vi "Is Transmit Ready.vi"(6 "Buffer size":i32=16384 format="0x%x (0d%d)", 8 "error in (no error)":errorcluster, 10 "Samples to transmit":i32=1024, 11 "Spectrum Recorder too in":refnum<class "Spectrum Recorder too.lvclass">) -> (0 "error out":errorcluster, 1 "Unused buffer":i32, 2 "Transmit Ready":bool, 3 "Spectrum Recorder too out":refnum<class "Spectrum Recorder too.lvclass">)   [LabVIEW 2016, in "Spectrum Recorder too.lvclass"]
uses:
  Spectrum Recorder too.lvclass
  Read RP transceiver.vi
  Write RP transceiver.vi
  NHMFL_Core/Libraries/Red Pitaya/RP Core/RP Transceiver/RP Transceiver.lvclass
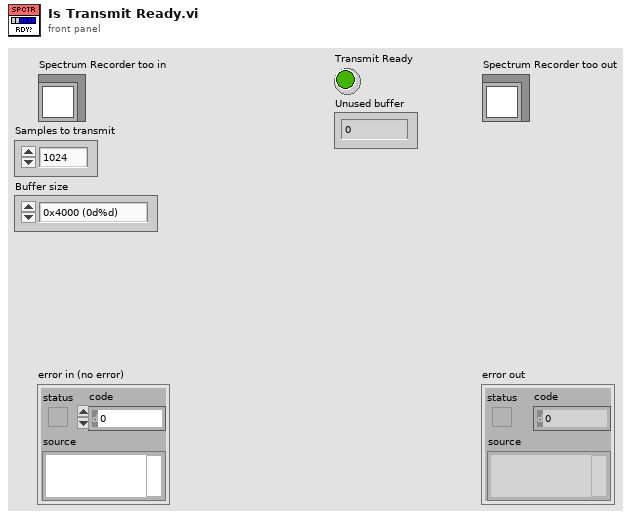
[diagram p1: front panel]
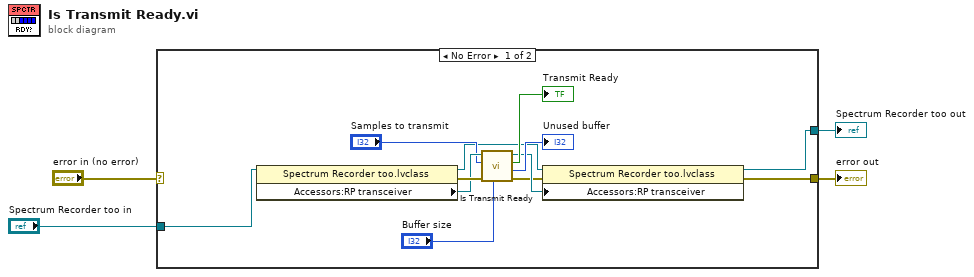
[diagram p0: block diagram]
diagram:
  n1 = case shown="No Error" "error in (no error)" {
    selector: "error in (no error)" -> [_ w18]
    tunnel: [w5 w18] -> w3
    tunnel: [w8 w17] -> w1
    tunnel: "Spectrum Recorder too in" -> [w15 w17]
    frame No Error {
      n2 = property class="Spectrum Recorder too.lvclass"(reference=w15) -> (reference out=w9:refnum<class "Spectrum Recorder too.lvclass">, error out=w16:errorcluster, "Accessors:RP transceiver"=w14:refnum<class "RP Transceiver.lvclass">)  [unwired: 1 in]
      n3 = call-dynamic "Is Transmit Ready.vi"("Buffer size"="Buffer size", "error in (no error)"=w16, "Samples to transmit"="Samples to transmit", "RP Instrument in"=w14) -> ("error out"=w6:errorcluster, "Unused buffer"=→"Unused buffer":i32, "Transmit Ready"=→"Transmit Ready":bool, "RP Instrument out"=w7:refnum<class "RP Transceiver.lvclass">)  [unwired: 4 in]
      n4 = property class="Spectrum Recorder too.lvclass"(reference=w9, error in=w6, "Accessors:RP transceiver"=w7) -> (reference out=w8:refnum<class "Spectrum Recorder too.lvclass">, error out=w5:errorcluster)
    }
    frame Error {
    }
  }
  "error out" <- w3
  "Spectrum Recorder too out" <- w1
